vi "(SubVI)_PID_AoWrite_Multivessels_for_test.vi"(0 "task in":refnum<k21>, 3 "amplitude":dbl=1.0 format="%0.2p", 5 "Filtered Dpp":dbl[](array[numeric]), 7 "Package from Galvo Pattern Generator":T3={"Freq of Stim. Pulse"=10.0, "sampling info"={"Fs"=1000.0, "#s"=1000.0}, "Galvo pattern"=[]} {"sampling info"."Fs" format="%.2p"; "Freq of Stim. Pulse" format="%0.2p"}, 9 "KpKiKdEi":T1, 11 "error in":errorcluster, 12 "Desired flow signal":dbl[](array[numeric])) -> (2 "Array":T2(array[cluster]), 4 "task out":refnum<k21>, 6 "DutyCycle (Display)":T4(graph), 8 "output KpKiKdEi":cluster{"Kp":dbl[], "Ki":dbl[], "Kd":dbl[]}, 10 "DutyCycleArray":dbl[](array[numeric]), 13 "Ed_out":dbl[](array[numeric]), 14 "Ei_out":dbl[](array[numeric]), 15 "error out":errorcluster)   [LabVIEW 2019]
uses:
  <vilib>/DAQmx/write.llb/DAQmx Write (Analog 2D DBL NChan NSamp).vi
  <vilib>/DAQmx/miscellaneous.llb/DAQmx Fill In Error Info.vi
  <vilib>/measure/NI_MABase.lvlib
panel:
  # "The first signal is placed at the begging of the concatenated signal"
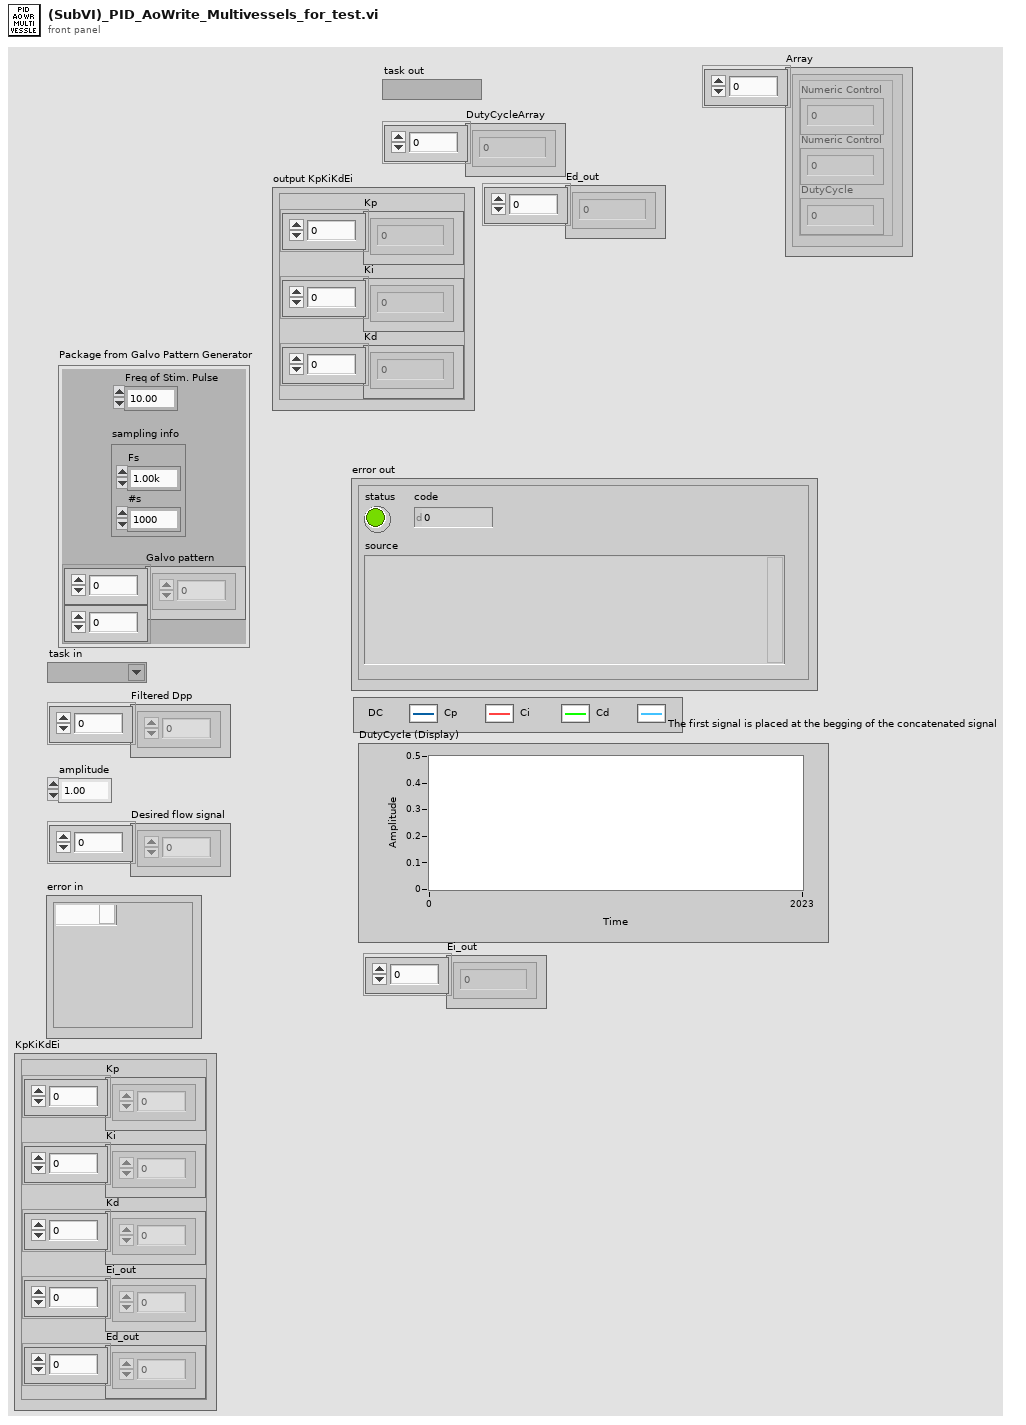
[diagram p1: front panel]
types:
  T1 = cluster{"Kp":dbl[], "Ki":dbl[], "Kd":dbl[], "Ei_out":dbl[], "Ed_out":dbl[]}
  T2 = cluster{"Numeric Control":dbl, "Numeric Control":dbl, "DutyCycle":dbl}[]
  T3 = cluster{"Freq of Stim. Pulse":dbl, "sampling info":cluster{"Fs":dbl, "#s":dbl}, "Galvo pattern":dbl[][]}
  T4 = cluster{"DutyCycle":dbl, "Cp":dbl, "Ci":dbl, "Cd":dbl}[]
  T5 = enum16{"Sine Wave", "Triangle Wave", "Square Wave", "Sawtooth Wave"}
  T6 = cluster{"DutyCycle":dbl, "Cp":dbl, "Ci":dbl, "Cd":dbl}
  T7 = cluster{"Numeric Control":dbl, "Numeric Control":dbl, "DutyCycle":dbl}
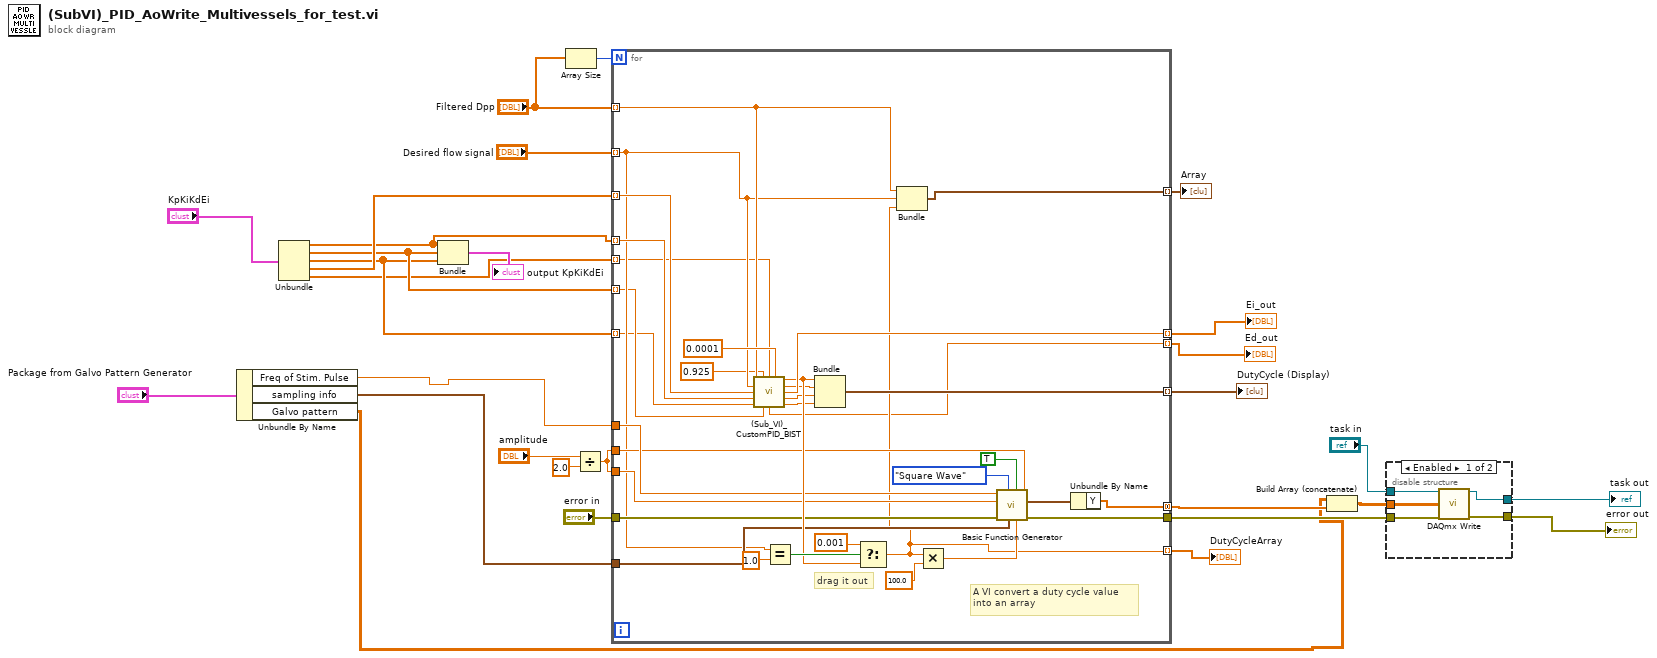
[diagram p0: block diagram]
diagram:
  n1 = Unbundle By Name("Package from Galvo Pattern Generator") -> ("Freq of Stim. Pulse"=w6:dbl, "sampling info"=w15:cluster{"Fs":dbl, "#s":dbl}, "Galvo pattern"=w5:dbl[][])
  n2 = Unbundle("KpKiKdEi") -> ("Kp"=w12:dbl[], "Ki"=w11:dbl[], "Kd"=w10:dbl[], "Ei_out"=w13:dbl[], "Ed_out"=w1:dbl[])
  n3 = Bundle("Kp"=w12, "Ki"=w11, "Kd"=w10) -> (→"output KpKiKdEi":cluster{"Kp":dbl[], "Ki":dbl[], "Kd":dbl[]})  [unwired: 1 in]
  n4 = Array Size(array="Filtered Dpp") -> (size(s)=w9:i32)
  n5 = Divide(x="amplitude", y=2.0) -> (x/y=w21:dbl)
  n6 = for {
    N: w9 -> [_]
    tunnel: "Desired flow signal" -> [w37] mode=indexing
    tunnel: "Filtered Dpp" -> [w38] mode=indexing
    tunnel: w13 -> [w62] mode=indexing
    tunnel: [w61] -> w29 mode=indexing
    tunnel: "error in" -> [w54]
    tunnel: w12 -> [w56] mode=indexing
    tunnel: w10 -> [w32] mode=indexing
    tunnel: w11 -> [w33] mode=indexing
    tunnel: [w55] -> w27 mode=indexing
    tunnel: w15 -> [w53]
    tunnel: w6 -> [w52]
    tunnel: w21 -> [w51]
    tunnel: [w50] -> w26
    tunnel: [w49] -> w8 mode=concatenating
    tunnel: w21 -> [w48]
    tunnel: [w36] -> w19 mode=indexing
    tunnel: [w35] -> w4 mode=indexing
    tunnel: [w31] -> w3 mode=indexing
    tunnel: w1 -> [w30] mode=indexing
    # "A VI convert a duty cycle value \ninto an array"
    # "drag it out"
    n7 = call "(Sub_VI)_CustomPID_BIST.vi"("Process Value"=w38, "Max Out"=0.925, "Ed_in"=w30, "Min Out"=0.0001, "Set Point"=w37, "Ei_in"=w62, "Kp"=w56, "Kd"=w32, "Ki"=w33) -> ("DutyCycle"=w57:dbl, "Cp"=w46:dbl, "Ei_out"=w61:dbl, "Ci"=w45:dbl, "Ed_out"=w31:dbl, "Cd"=w44:dbl)  [unwired: 1 in]
    n8 = Equal?(x=w37, y=1.0) -> (x = y?=w59:bool)
    n9 = Bundle("DutyCycle"=w57, "Cp"=w46, "Ci"=w45, "Cd"=w44) -> (w55:T6)  [unwired: 1 in]
    n10 = Select(t=0.001, s=w59, f=w57) -> (s? t:f=w36:dbl)
    n11 = Bundle("Numeric Control"=w38, "Numeric Control"=w37, "DutyCycle"=w36) -> (w35:T7)  [unwired: 1 in]
    n12 = Multiply(x=w36, y=100.0) -> (x*y=w41:dbl)
    n13 = call <vilib>:"Basic Function Generator.vi"("offset"=w48, "square wave duty cycle (%)"=w41, "reset signal"=TRUE, "sampling info"=w53, "signal type"=T5."Square Wave", "error in (no error)"=w54, "amplitude"=w51, "frequency"=w52) -> ("error out"=w50:errorcluster, "signal out"=w42:waveform(dbl))  [unwired: 1 in, 1 out]
    n14 = Unbundle By Name(w42) -> ("Y"=w49:dbl[])
  }
  "Ei_out" <- w29
  "DutyCycle (Display)" <- w27
  "DutyCycleArray" <- w19
  "Array" <- w4
  "Ed_out" <- w3
  n15 = Build Array (concatenate)(w5, w8) -> (w7:dbl[][])
  n16 = disable-structure shown="Enabled" {
    disable-tunnel: w26 -> [w67 _]
    disable-tunnel: "task in" -> [w66 _]
    disable-tunnel: [w65 _] -> w24
    disable-tunnel: [w64 _] -> w23
    disable-tunnel: w7 -> [w63 _]
    frame Enabled {
      n17 = call-poly <vilib>:"DAQmx Write.vi"("task/channels in"=w66, "data"=w63, "error in"=w67) -> ("task out"=w65:refnum<k21>, "error out"=w64:errorcluster)  [unwired: 10 in, 1 out]
    }
    frame Disabled {
    }
  }
  "task out" <- w24
  "error out" <- w23
